vi "LV SciSDK LIST.vi"(0 "Buffer Size":u32=1, 7 "List Handle In":cluster{"List Path":string, "List Name":string}, 9 "Board Handle In":T1, 11 "error in (no error)":errorcluster) -> (4 "NI Error Code":i32, 6 "List Buffer Out":T2, 8 "List Handle Out":cluster{"List Path":string, "List Name":string}, 10 "Board Handle Out":T1, 15 "error out":errorcluster)   [LabVIEW 2021, in "SciSDK_Labview.lvlib"]
doc: "You need this VI to read data from a list component"
uses:
  SciSDK_Labview.lvlib
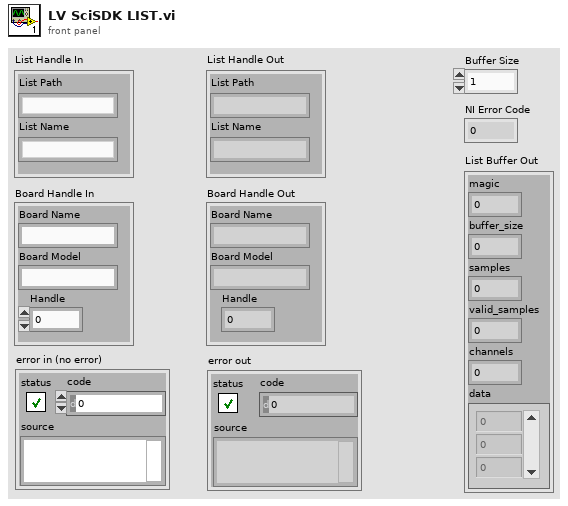
[diagram p1: front panel]
types:
  T1 = cluster{"Board Name":string, "Board Model":string, "Handle":u64}
  T2 = cluster{"magic":u32, "buffer_size":u32, "samples":u32, "valid_samples":u32, "channels":u32, "data":i8[]}
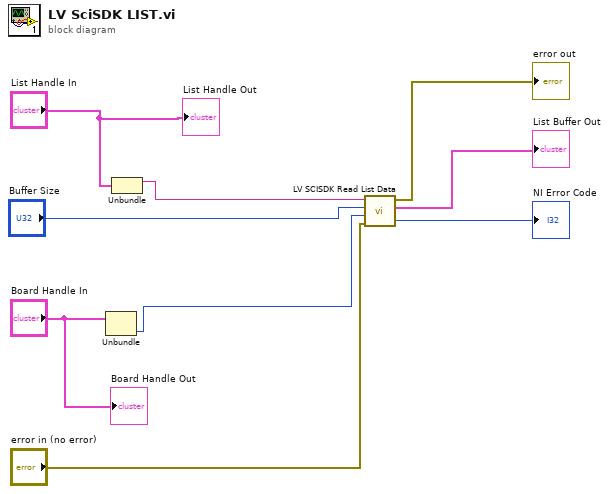
[diagram p0: block diagram]
diagram:
  n1 = Unbundle("Board Handle In") -> ("Handle"=w2:u64)  [unwired: 2 out]
  n2 = Unbundle("List Handle In") -> ("List Path"=w3:string)  [unwired: 1 out]
  n3 = call "LV SCISDK Read List Data.vi"("Path"=w3, "Buffer Size"="Buffer Size", "handle"=w2, "error in (no error)"="error in (no error)") -> ("error out"=→"error out":errorcluster, "buffer out"=→"List Buffer Out":T2, "function return"=→"NI Error Code":i32)  [unwired: 3 in, 1 out]
  "List Handle Out" <- "List Handle In"
  "Board Handle Out" <- "Board Handle In"
